vi "itemsLow.vi"(8 "error in (no error)":errorcluster, 11 "reference in":refnum<class "Project Panels.lvclass">=refnum) -> (0 "error out":errorcluster={"status"=TRUE, "code"=1556, "source"="In Place Element Structure in Project Panels.lvclass:items.vi"}, 2 "saved?":bool, 3 "reference out":refnum<class "Project Panels.lvclass">)   [LabVIEW 2015, in "Project Panels.lvclass"]
uses:
  Project Panels.lvclass
  SYS/Items Controller_llb/storageSheets.ctl
  stateItem.ctl
  <vilib>/Utility/miscctls.llb/LVRowAndColumnUnsignedTypeDef.ctl
  <vilib>/Utility/miscctls.llb/LVRowAndColumnTypeDef.ctl
  SYS/Items Controller_llb/Items Controller.lvclass
  SYS/File Controller_llb/File Controller.lvclass
panel:
  out "title":string="Cosmed Asia Pacific - Storage"
  in  "tables":enum32{"Check IN", "Check OUT", "Storage"}(tab)
  in  "checkIN":string[][](table)
  in  "checkOUT":string[][](table)
  in  "Storage":string[][](table)
  in  "uploadFile":bool
  in  "Add Check OUT":bool
  in  "Add Check IN":bool
  out "Number of Items:":i32
  out "index":i32
  in  "back":bool
  in  "next":bool
  out "storageSheets":T1
  in  "Search Item":bool
  in  "Save":bool
  out "Item Selected (S/N or P/N):":string
  out "statuBar":string="Stoped for an Error"
  in  "Stop Button":bool
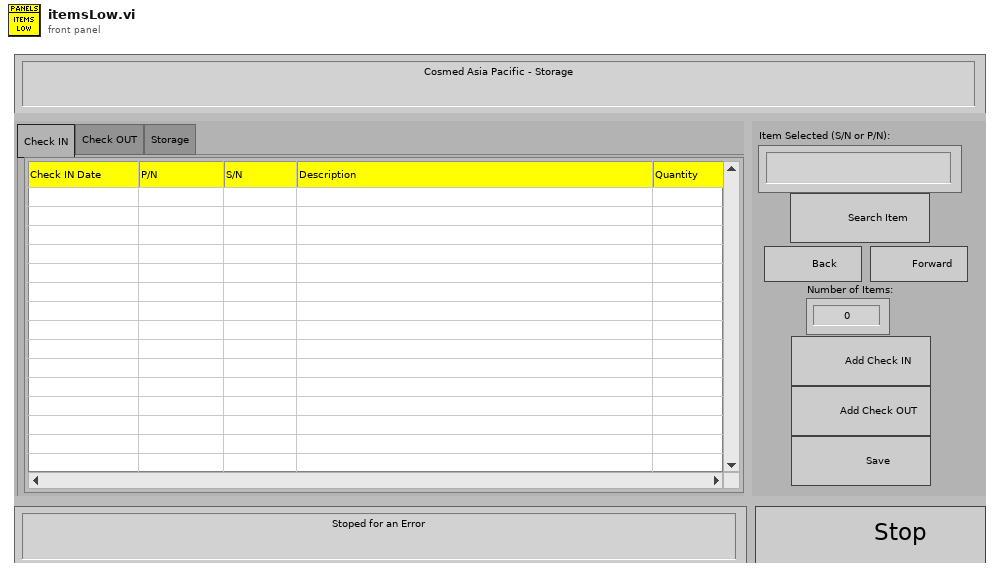
[diagram p1: front panel]
types:
  T1 = typedef "Items Controller.lvclass/storageSheets.ctl" = enum16{"check-in", "check-out", "storage"}
  T2 = typedef "Project Panels.lvclass/stateItem.ctl" = enum16{"initiate", "waitEvent", "save", "search", "UploadFile", "nextItems", "stop"}
  T3 = typedef "LVRowAndColumnUnsignedTypeDef.ctl" = cluster{"Row":u32, "Column":u32}
  T4 = enum8{"Enabled", "Disabled", "Disabled and Grayed Out"}
  T5 = cluster{"checkIN":string[][], "checkOUT":string[][], "storage":string[][]}
  T6 = typedef "LVRowAndColumnTypeDef.ctl" = cluster{"Row":i32, "Column":i32}
  T7 = typedef "Project Panels.lvclass/ObjectAttributesRef.ctl" = refnum<data-value>
  T8 = typedef "Project Panels.lvclass/ObjectAttributes.ctl" = cluster{"MyAttribute":dbl, "device_controller_ref":refnum<class "Devices Controller.lvclass">, "file_controller_ref":refnum<class "File Controller.lvclass">, "item_controller_ref":refnum<class "Items Controller.lvclass">, "item_tables":cluster{"checkIN":string[][], "checkOUT":string[][], "storage":string[][]}, "quickbook_table":cluster{"notes":string[][]}, "notification_controller_ref":refnum<class "Notification Controller.lvclass">, "partstracking_controller_ref":refnum<class "PartsTracking Controller.lvclass">, "product_tables":cluster{"k4b2":string[][], "fitmate":string[][], "RMR":string[][], "CPET":string[][], "BP":string[][], "PP":string[][], "k5":string[][], "bb-pft":string[][]}, "rowsColour":u32[], "low_resolution?":bool, "run_python?":bool}
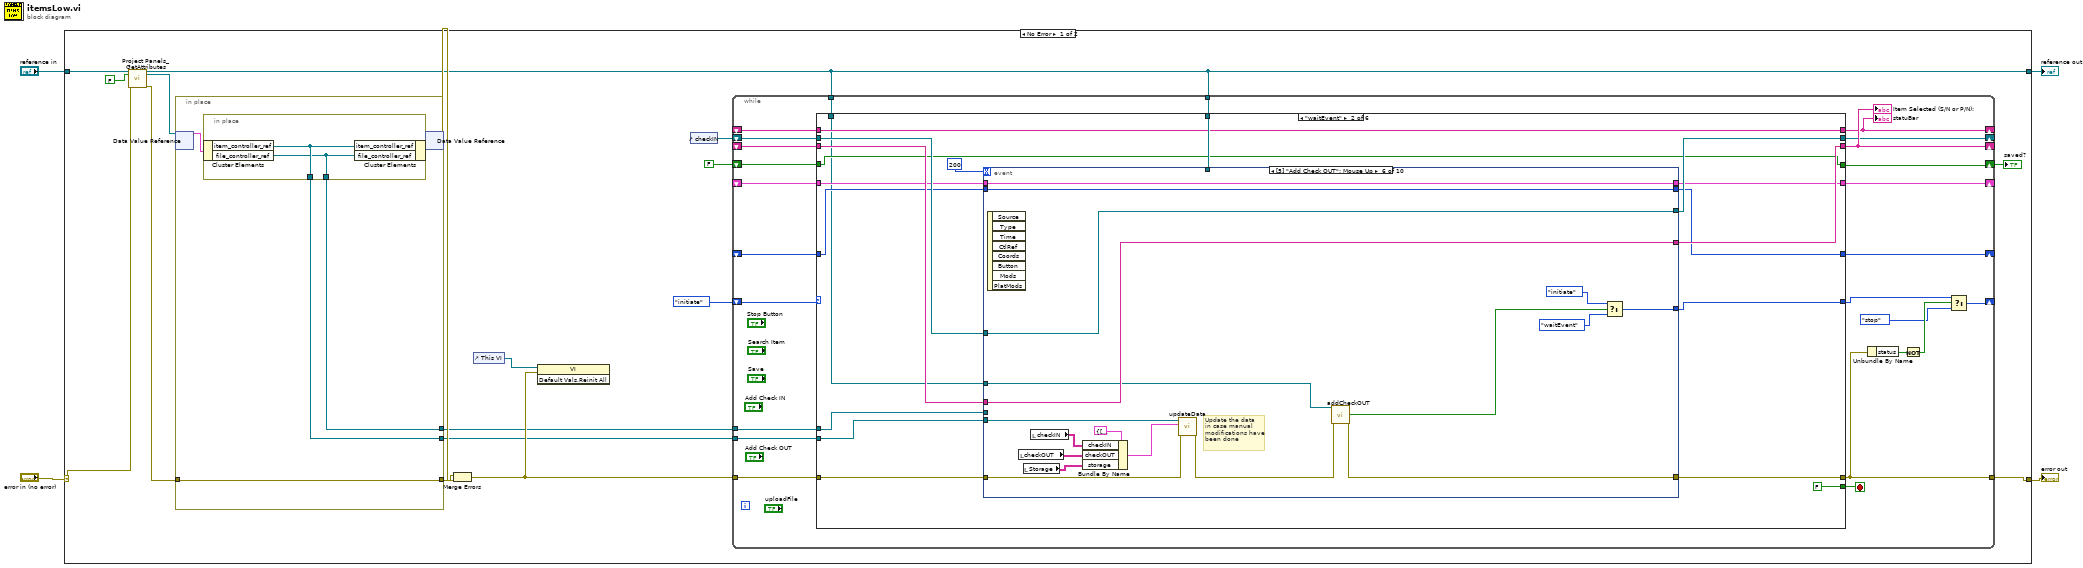
[diagram p0: block diagram]
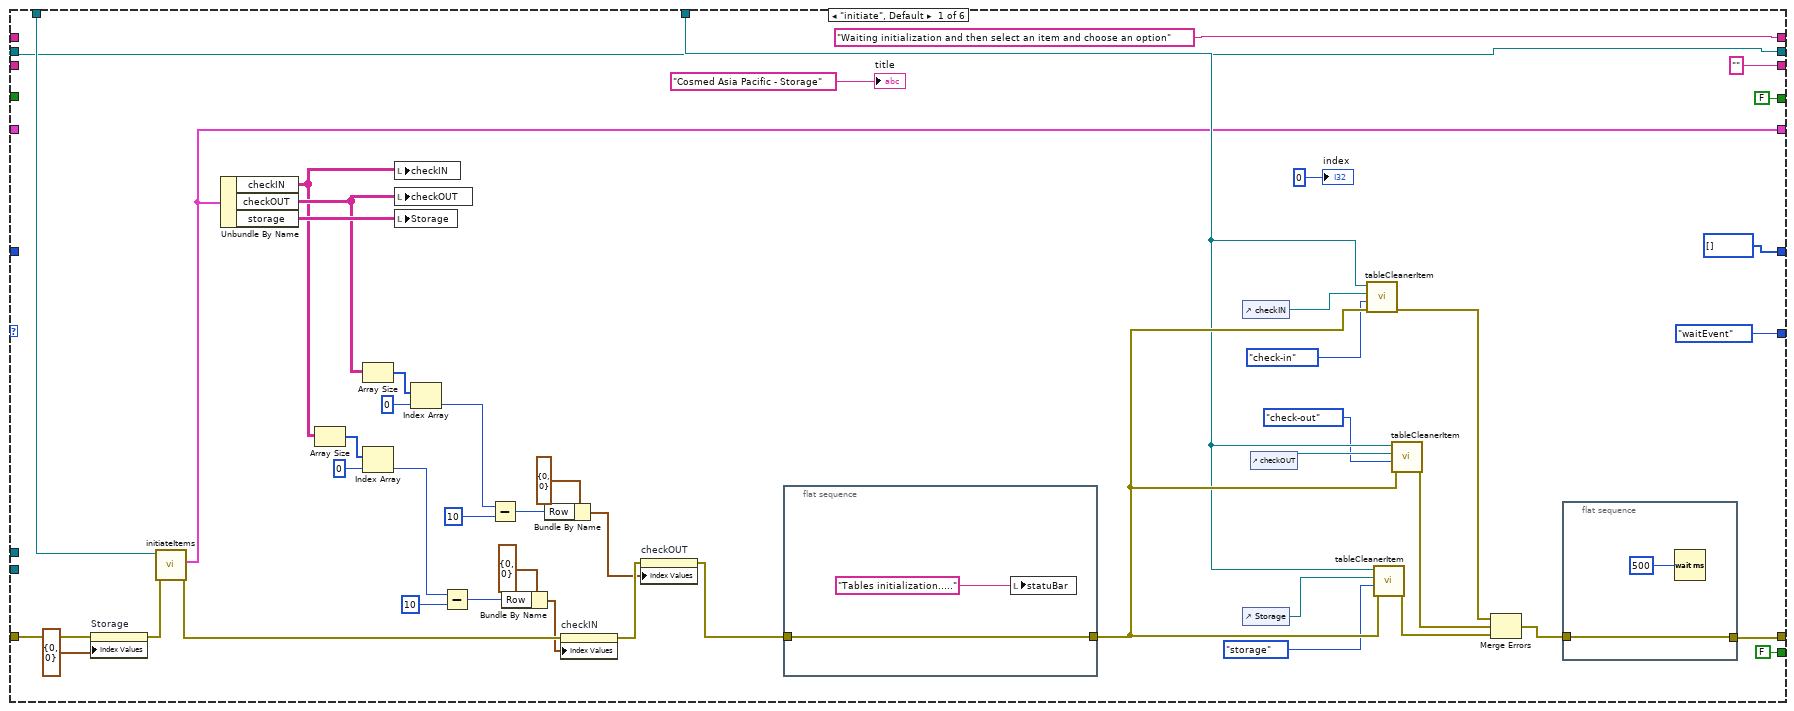
[diagram p2: hidden frame]
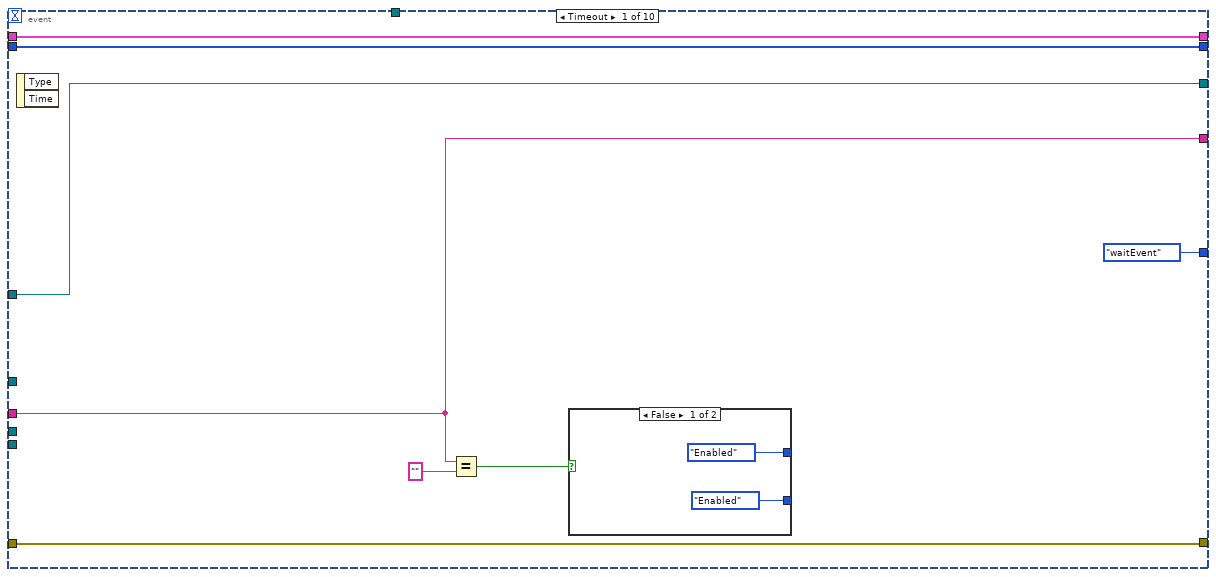
[diagram p3: hidden frame]
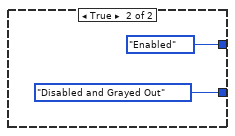
[diagram p4: hidden frame]
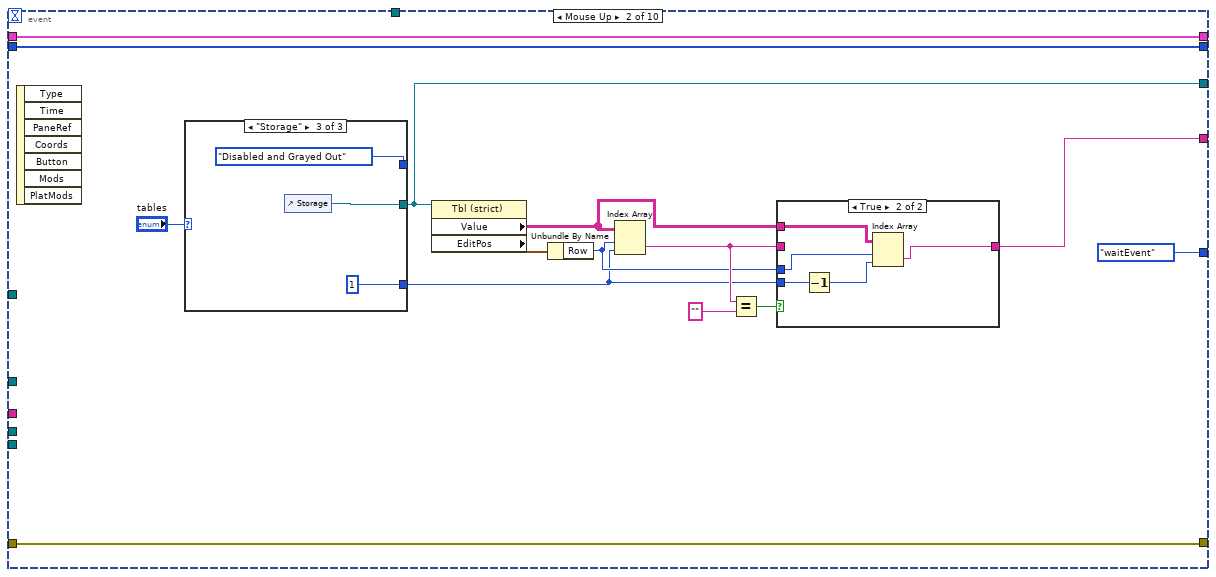
[diagram p5: hidden frame]
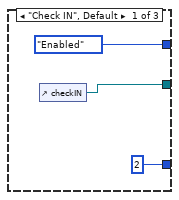
[diagram p7: hidden frame]
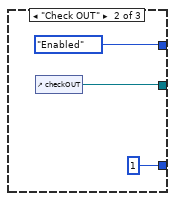
[diagram p8: hidden frame]
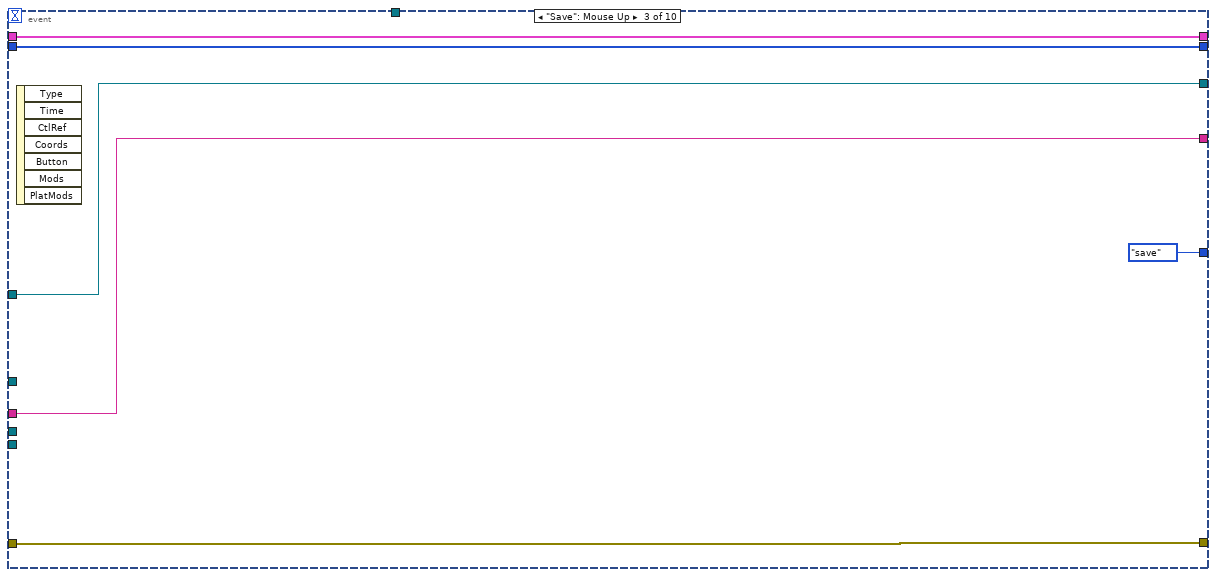
[diagram p9: hidden frame]
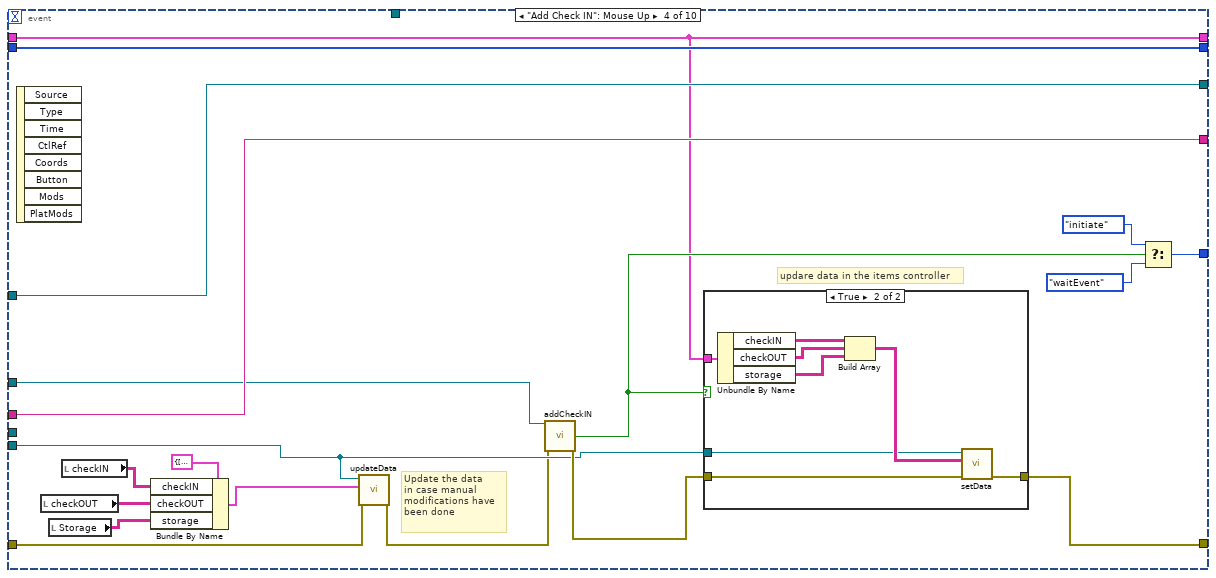
[diagram p10: hidden frame]
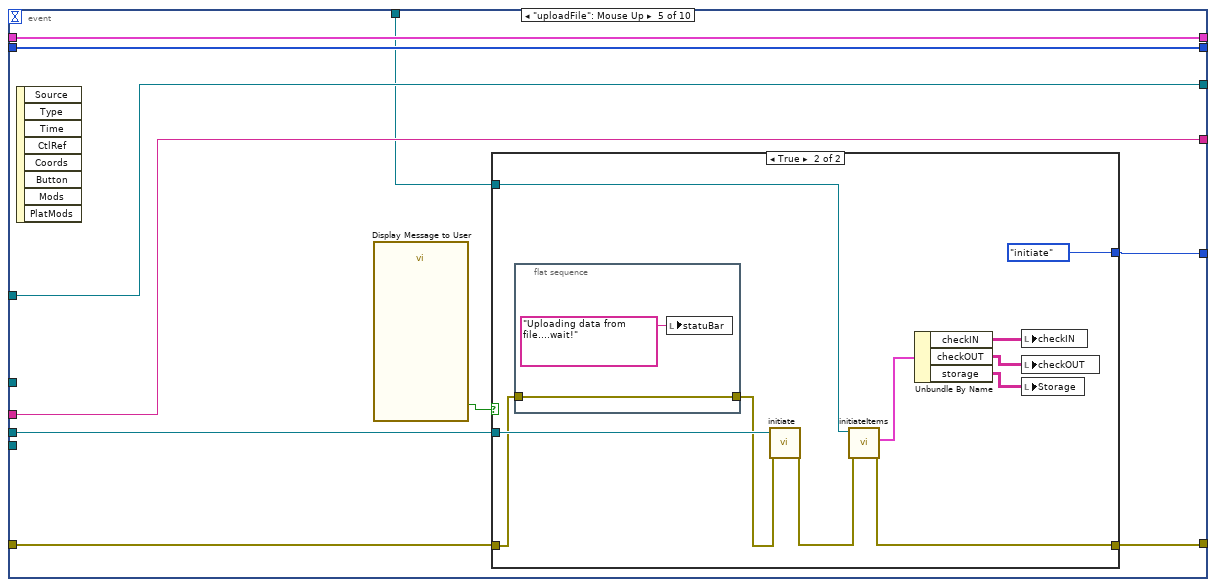
[diagram p12: hidden frame]
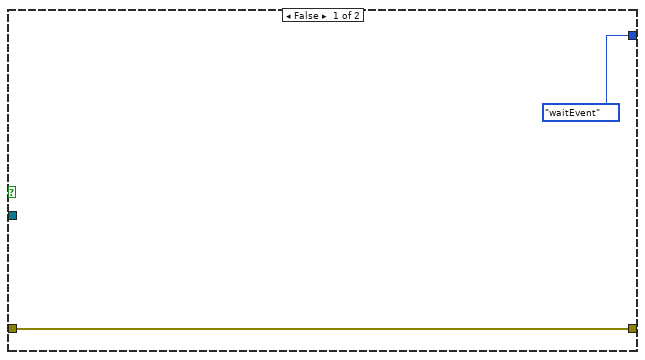
[diagram p13: hidden frame]
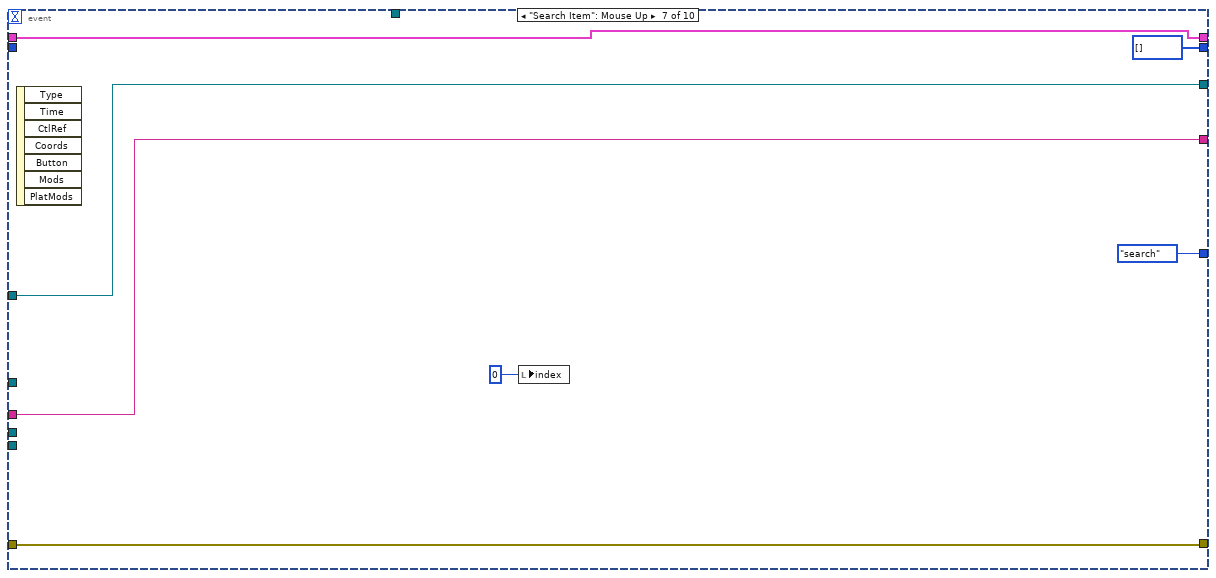
[diagram p14: hidden frame]
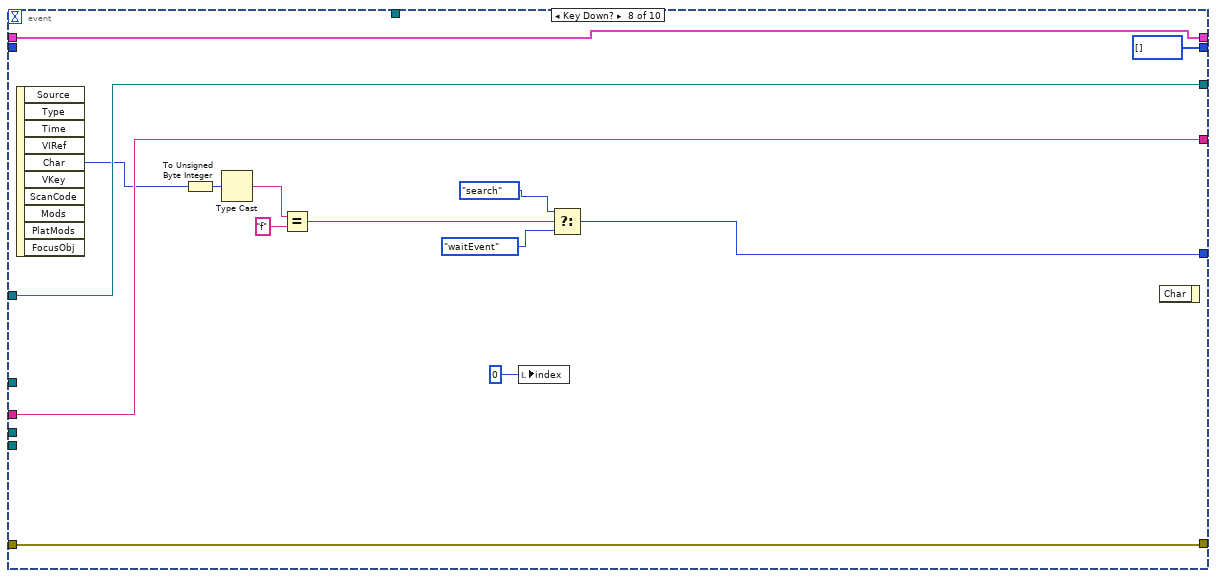
[diagram p15: hidden frame]
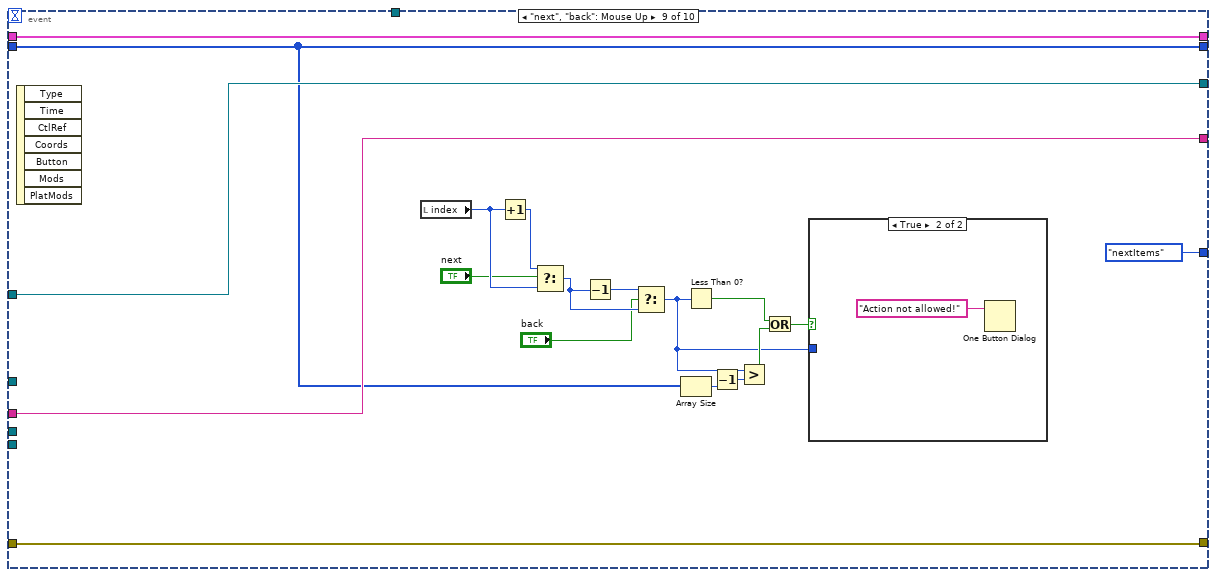
[diagram p16: hidden frame]
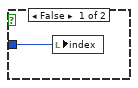
[diagram p17: hidden frame]
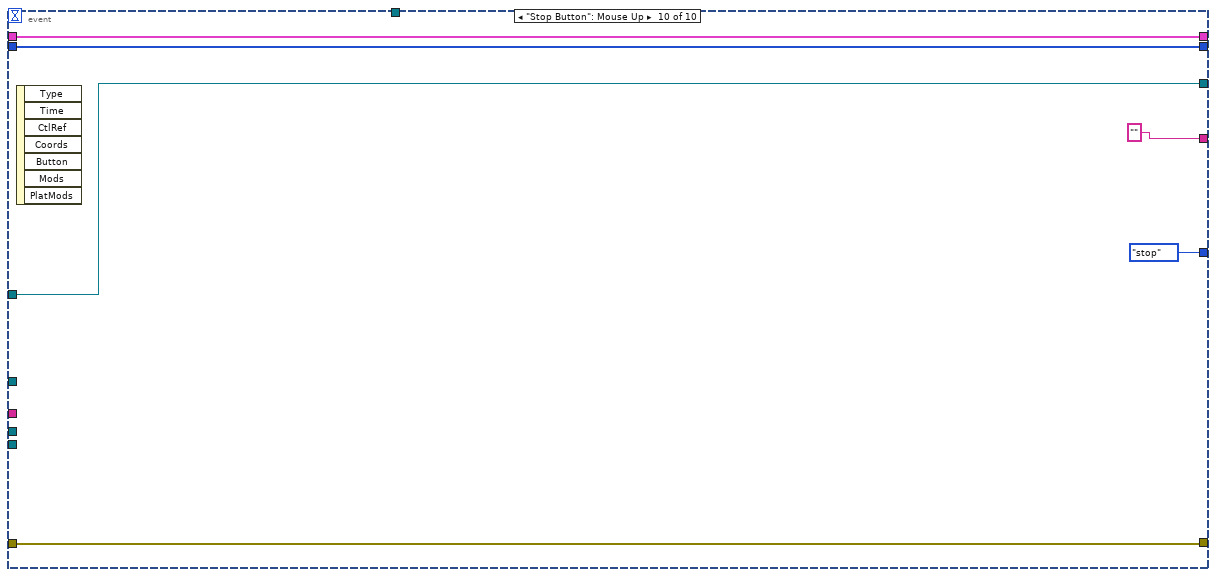
[diagram p18: hidden frame]
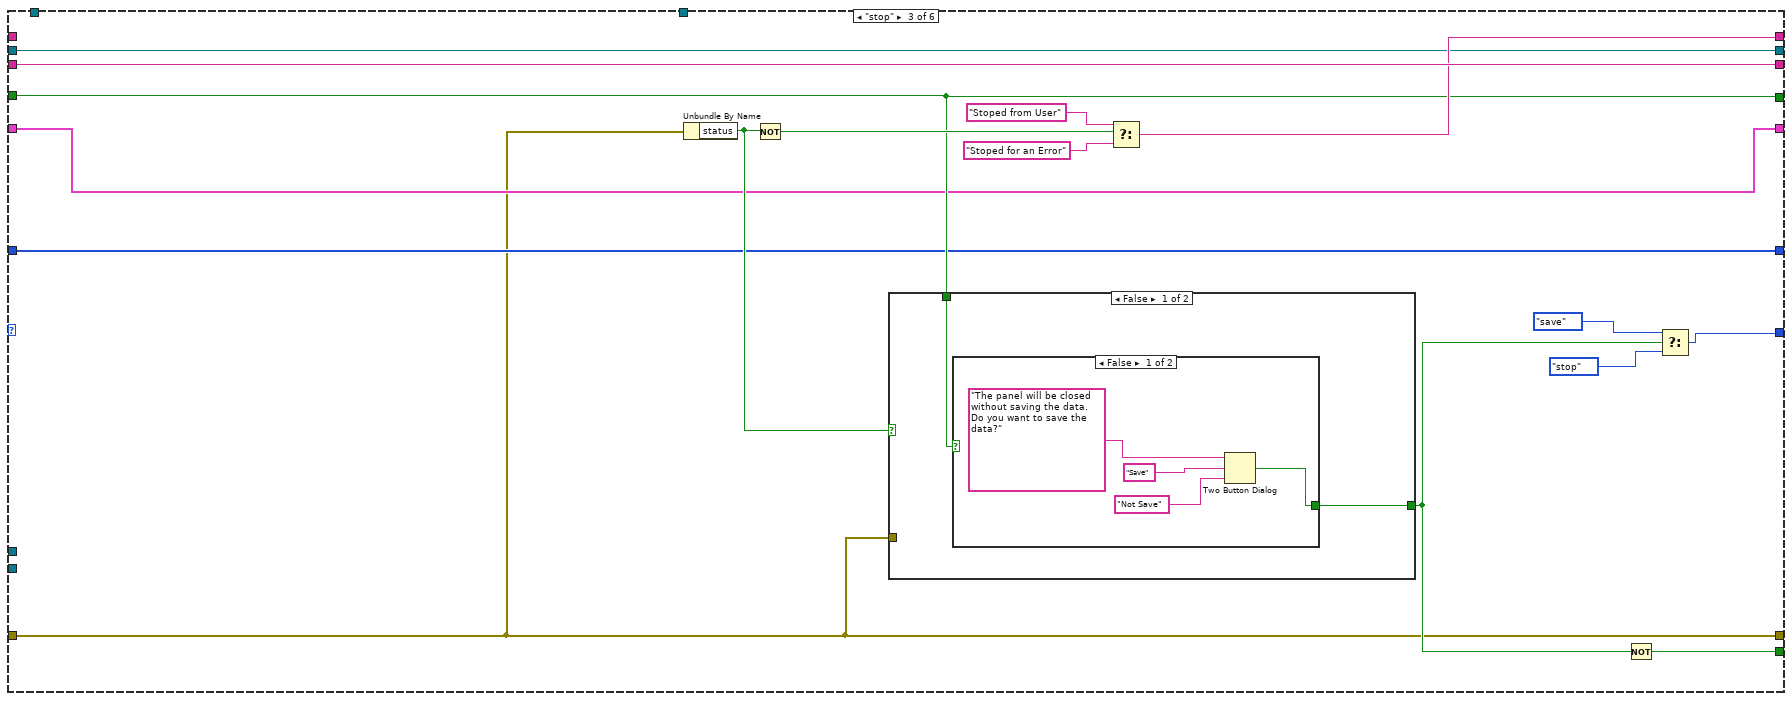
[diagram p19: hidden frame]
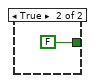
[diagram p20: hidden frame]
diagram:
  n1 = case shown="No Error" "error in (no error)" {
    selector: "error in (no error)" -> [w17 w412]
    tunnel: [w14 w412] -> w3
    tunnel: [w12 w411] -> w1
    tunnel: "reference in" -> [w19 w411]
    frame No Error {
      n2 = call "Project Panels_GetAttributes.vi"("reference in"=w19, "return data? (T)"=FALSE, "error in (no error)"=w17) -> ("reference out"=w12:refnum<class "Project Panels.lvclass">, "attributes ref"=w15:T7, "error out"=w16:errorcluster)  [unwired: 13 in, 1 out]
      n3 = in-place {
        in-place-border: w16 -> [w406]
        in-place-border: [w406] -> w20
        in-place-border: [w405] -> w8
        in-place-border: [w404] -> w5
        n4 = in-place-dvr #1(w15) -> (w407:T8)  [unwired: 1 out]
        n5 = in-place {
          in-place-border: [w410] -> w405
          in-place-border: [w409] -> w404
          n6 = in-place-cluster #2(w407) -> ("item_controller_ref"=w410:refnum<class "Items Controller.lvclass">, "file_controller_ref"=w409:refnum<class "File Controller.lvclass">)
          n7 = in-place-cluster #2("item_controller_ref"=w410, "file_controller_ref"=w409) -> (w408:T8)
        }
        n8 = in-place-dvr #1(w408) -> (w21:errorcluster)  [unwired: 1 out]
      }
      n9 = Merge Errors(w20, w21) -> (w9:errorcluster)
      n10 = control-ref of="This VI"() -> (w10:refnum<vi>)
      n11 = invoke class="VI" method="Default Vals.Reinit All"(reference=w10, error in=w9) -> ()  [unwired: 1 in, 3 out]
      n12 = control-ref of="checkIN"() -> (w11:refnum<vi>)
      n13 = while {
        tunnel: w12 -> [w46]
        tunnel: w9 -> [w45]
        tunnel: [w43] -> w14
        shift-right: [w40] -> _
        shift-left: stateItem."initiate" ("state") -> [w44]
        shift-right: [w37] -> _
        shift-left: _ -> [w36]
        shift-right: [w35] -> _
        shift-left: w11 -> [w34]
        tunnel: w12 -> [w33]
        tunnel: w8 -> [w31]
        shift-right: [w29] -> w6
        shift-left: FALSE -> [w30]
        shift-right: [w28] -> _
        shift-left: _ -> [w27]
        shift-right: [w26] -> _
        shift-left: _ -> [w25]
        shift-right: [w24] -> _
        shift-left: _ -> [w23]
        tunnel: w5 -> [w22]
        stop <- w38 stop-if-true
        n14 = case shown="\"waitEvent\"" w44 {
          tunnel: w46 -> [w81 w106 _ _ _ _]
          tunnel: w45 -> [w74 w115 w282 w310 w342 w377]
          tunnel: [w84 w109 w282 w321 w342 w373] -> w43
          tunnel: [stateItem."waitEvent" ("state") w108 w288 w316 stateItem."waitEvent" ("state") stateItem."waitEvent" ("state")] -> w41
          tunnel: [FALSE FALSE w287 FALSE FALSE FALSE] -> w38
          tunnel: ["Waiting initialization and then select an item and choose an option" ("title") w104 w294 "Search Item option selected..." ("title") "Click on the arrows to select other items" ("title") w372] -> w28
          tunnel: ["" w111 w297 w322 w339 w378] -> w37
          tunnel: w36 -> [_ w113 w297 w322 w339 w378]
          tunnel: [w78 w110 w293 w323 w333 w379] -> w35
          tunnel: w34 -> [w78 w112 w293 w323 w333 w379]
          tunnel: w33 -> [w80 w99 _ w312 _ _]
          tunnel: w31 -> [_ w107 _ _ _ w350]
          tunnel: w30 -> [_ w105 w286 w320 w340 _]
          tunnel: [FALSE w105 w286 w320 w340 TRUE] -> w29
          tunnel: w27 -> [_ w104 _ _ _ _]
          tunnel: [i32[] [] ("indexElements") w102 w285 w314 w334 w375] -> w26
          tunnel: w25 -> [_ w103 w285 _ w334 w375]
          tunnel: [w47 w100 w284 w311 w326 w371] -> w24
          tunnel: w23 -> [_ w101 w284 w311 w326 w371]
          tunnel: w22 -> [_ w98 _ _ _ _]
          frame "initiate", Default {
            n15 = property on="Storage" class="Tbl (strict)"(error in=w74, "Index Values"=T3 {"Row"=0, "Column"=0}) -> (error out=w73:errorcluster)  [unwired: 1 in, 1 out]
            n16 = call "initiateItems.vi"("error in (no error)"=w73, "reference in"=w80) -> ("error out"=w65:errorcluster, "table"=w47:T5)  [unwired: 7 in, 1 out]
            n17 = Unbundle By Name(w47) -> ("checkIN"=w48:string[][], "checkOUT"=w67:string[][], "storage"=w72:string[][])
            n18 = Array Size(array=w48) -> (size(s)=w54:i32[])
            n19 = Array Size(array=w67) -> (size(s)=w61:i32[])
            n20 = Index Array(array=w54, index=0) -> (element=w51:i32)
            n21 = local write "checkIN"(w48) -> ()
            n22 = local write "checkOUT"(w67) -> ()
            n23 = local write "Storage"(w72) -> ()
            n24 = Index Array(array=w61, index=0) -> (element=w58:i32)
            n25 = Subtract(x=w51, y=10) -> (x-y=w52:i32)
            n26 = Subtract(x=w58, y=10) -> (x-y=w59:i32)
            n27 = Bundle By Name(cluster=T3 {"Row"=0, "Column"=0} ("Index Values"), "Row"=w52) -> (w49:T3)
            n28 = Bundle By Name(cluster=T3 {"Row"=0, "Column"=0} ("Index Values"), "Row"=w59) -> (w56:T3)
            n29 = property on="checkIN" class="Tbl (strict)"(error in=w65, "Index Values"=w49) -> (error out=w64:errorcluster)  [unwired: 1 in, 1 out]
            n30 = property on="checkOUT" class="Tbl (strict)"(error in=w64, "Index Values"=w56) -> (error out=w66:errorcluster)  [unwired: 1 in, 1 out]
            n31 = flat-sequence {
              tunnel: w66 -> [w95]
              tunnel: [w95] -> w83
              frame #0 {
                n32 = local write "statuBar"("Tables initialization....." ("title")) -> ()
              }
            }
            n33 = control-ref of="checkIN"() -> (w91:refnum<vi>)
            n34 = control-ref of="Storage"() -> (w93:refnum<vi>)
            n35 = control-ref of="checkOUT"() -> (w92:refnum<vi>)
            n36 = call "tableCleanerItem.vi"("error in (no error)"=w83, "storageSheets"=storageSheets."check-in", "Table in"=w91, "reference in"=w81) -> ("error out"=w90:errorcluster)  [unwired: 6 in, 1 out]
            n37 = call "tableCleanerItem.vi"("error in (no error)"=w83, "storageSheets"=storageSheets."storage", "Table in"=w93, "reference in"=w81) -> ("error out"=w88:errorcluster)  [unwired: 6 in, 1 out]
            n38 = call "tableCleanerItem.vi"("error in (no error)"=w83, "storageSheets"=storageSheets."check-out", "Table in"=w92, "reference in"=w81) -> ("error out"=w89:errorcluster)  [unwired: 6 in, 1 out]
            n39 = Merge Errors(w90, w89, w88) -> (w79:errorcluster)
            n40 = flat-sequence {
              tunnel: w79 -> [w97]
              tunnel: [w97] -> w84
              frame #0 {
                n41 = Wait (ms)(milliseconds to wait=u32 500) -> ()  [unwired: 1 out]
              }
            }
            "title" <- "Cosmed Asia Pacific - Storage" ("title")
            "index" <- 0 ("index")
          }
          frame "waitEvent" {
            n42 = event shown="[5] \"Add Check OUT\": Mouse Up" {
              selector: _ -> [_ _ _ _ _ _ _ _ _ _]
              dyn-events: _ -> [_ _ _ _ _ _ _ _ _ _]
              timeout: 200 -> [_ _ _ _ _ _ _ _ _ _]
              tunnel: w115 -> [w124 w142 w158 w170 w197 w225 w238 w253 w273 w281]
              tunnel: [w124 w142 w158 w173 w196 w230 w238 w253 w273 w281] -> w109
              tunnel: w113 -> [w120 _ w162 w182 w198 w234 w240 w254 w266 _]
              tunnel: w112 -> [w121 _ w163 w181 w199 w233 w241 w255 w267 w279]
              tunnel: [w120 w135 w162 w182 w198 w234 w240 w254 w266 ""] -> w111
              tunnel: [w121 w139 w163 w181 w199 w233 w241 w255 w267 w279] -> w110
              tunnel: [stateItem."waitEvent" ("state") stateItem."waitEvent" ("state") stateItem."save" ("state") w177 w194 w228 stateItem."search" ("state") w243 stateItem."nextItems" ("state") stateItem."stop" ("state")] -> w108
              tunnel: w107 -> [_ _ _ w172 _ w223 _ _ _ _]
              tunnel: w106 -> [_ _ _ _ w192 _ _ _ _ _]
              tunnel: w103 -> [w118 w130 w160 w180 w200 w232 _ _ w265 w277]
              tunnel: [w118 w130 w160 w180 w200 w232 i32[] [] ("indexElements") i32[] [] ("indexElements") w265 w277] -> w102
              tunnel: w101 -> [w117 w129 w159 w171 w201 w222 w235 w250 w256 w276]
              tunnel: [w117 w129 w159 w171 w201 w222 w235 w250 w256 w276] -> w100
              tunnel: w99 -> [_ _ _ w179 _ w231 _ _ _ _]
              tunnel: w98 -> [_ _ _ _ w193 _ _ _ _ _]
              event Timeout {
                n43 = event-data() -> ()  [unwired: 1 in, 2 out]
                n44 = Equal?(x=w120, y="") -> (x = y?=w123:bool)
                n45 = case shown="False" w123 {
                  tunnel: [T4."Enabled" ("Disabled") T4."Disabled and Grayed Out" ("Disabled")] -> _
                  tunnel: [T4."Enabled" ("Disabled") T4."Enabled" ("Disabled")] -> _
                  frame False {
                  }
                  frame True {
                  }
                }
              }
              event Mouse Up {
                n46 = event-data() -> ()  [unwired: 1 in, 7 out]
                n47 = case shown="\"Storage\"" "tables" {
                  tunnel: [w151 w154 w157] -> w139
                  tunnel: [T4."Enabled" ("Disabled") T4."Enabled" ("Disabled") T4."Disabled and Grayed Out" ("Disabled")] -> _
                  tunnel: [2 ("disabled index (col)") 1 ("disabled index (col)") 1 ("disabled index (col)")] -> w132
                  frame "Check IN", Default {
                    n48 = control-ref of="checkIN"() -> (w151:refnum<vi>)
                  }
                  frame "Check OUT" {
                    n49 = control-ref of="checkOUT"() -> (w154:refnum<vi>)
                  }
                  frame "Storage" {
                    n50 = control-ref of="Storage"() -> (w157:refnum<vi>)
                  }
                }
                n51 = property on="Property Node" class="Tbl (strict)"(reference=w139) -> ("Value"=w134:string[][], "EditPos"=w141:T6)  [unwired: 1 in, 2 out]
                n52 = Unbundle By Name(w141) -> ("Row"=w133:i32)
                n53 = Index Array(array=w134, index (row)=w133, index (col)=w132) -> (element=w136:string)
                n54 = Equal?(x=w136, y="") -> (x = y?=w137:bool)
                n55 = case shown="True" w137 {
                  tunnel: w136 -> [w143 _]
                  tunnel: [w143 w144] -> w135
                  tunnel: w134 -> [_ w148]
                  tunnel: w133 -> [_ w147]
                  tunnel: w132 -> [_ w146]
                  frame False {
                  }
                  frame True {
                    n56 = Decrement(x=w146) -> (x-1=w145:i32)
                    n57 = Index Array(array=w148, index (row)=w147, index (col)=w145) -> (element=w144:string)
                  }
                }
              }
              event "Save": Mouse Up {
                n58 = event-data() -> ()  [unwired: 1 in, 7 out]
              }
              event "Add Check IN": Mouse Up {
                # "Update the data\nin case manual\nmodifications have\nbeen done"
                # "updare data in the items controller"
                n59 = event-data() -> ()  [unwired: 1 in, 8 out]
                n60 = local read "checkOUT"() -> (w166:string[][])
                n61 = local read "Storage"() -> (w165:string[][])
                n62 = local read "checkIN"() -> (w167:string[][])
                n63 = Bundle By Name(cluster=T5 {"checkIN"=[], "checkOUT"=[], "storage"=[]} ("table"), "checkIN"=w167, "checkOUT"=w166, "storage"=w165) -> (w164:T5)
                n64 = call "updateData.vi"("error in (no error)"=w170, "table"=w164, "reference in"=w172) -> ("error out"=w169:errorcluster)  [unwired: 7 in, 1 out]
                n65 = call "addCheckIN.vi"("reference in"=w179, "error in (no error)"=w169) -> ("saved?"=w175:bool, "error out"=w174:errorcluster)  [unwired: 11 in, 1 out]
                n66 = case shown="True" w175 {
                  tunnel: w171 -> [_ w187]
                  tunnel: w174 -> [w183 w186]
                  tunnel: [w183 w185] -> w173
                  tunnel: w172 -> [_ w184]
                  frame False {
                  }
                  frame True {
                    n67 = Unbundle By Name(w187) -> ("checkIN"=w191:string[][], "checkOUT"=w190:string[][], "storage"=w189:string[][])
                    n68 = Build Array(w191, w190, w189) -> (w188:string[][][])
                    n69 = call "setData.vi"("error in (no error)"=w186, "data"=w188, "reference in"=w184) -> ("error out"=w185:errorcluster)  [unwired: 7 in, 1 out]
                  }
                }
                n70 = Select(t=stateItem."initiate" ("state"), s=w175, f=stateItem."waitEvent") -> (s? t:f=w177:T2)
              }
              event "uploadFile": Mouse Up {
                n71 = event-data() -> ()  [unwired: 1 in, 8 out]
                n72 = call "Display Message to User"() -> ("Yes"=w195:bool)  [unwired: 10 in, 1 out]
                n73 = case shown="True" w195 {
                  tunnel: w197 -> [w203 w205]
                  tunnel: [w203 w209] -> w196
                  tunnel: [stateItem."waitEvent" ("state") stateItem."initiate" ("state")] -> w194
                  tunnel: w193 -> [_ w213]
                  tunnel: w192 -> [_ w211]
                  frame False {
                  }
                  frame True {
                    n74 = flat-sequence {
                      tunnel: w205 -> [w216]
                      tunnel: [w216] -> w204
                      frame #0 {
                        n75 = local write "statuBar"("Uploading data from file....wait!" ("statuBar")) -> ()
                      }
                    }
                    n76 = call "initiate.vi"("reference in"=w213, "error in (no error)"=w204) -> ("error out"=w210:errorcluster)  [unwired: 16 in, 1 out]
                    n77 = call "initiateItems.vi"("error in (no error)"=w210, "reference in"=w211) -> ("error out"=w209:errorcluster, "table"=w212:T5)  [unwired: 7 in, 1 out]
                    n78 = Unbundle By Name(w212) -> ("checkIN"=w208:string[][], "checkOUT"=w207:string[][], "storage"=w206:string[][])
                    n79 = local write "checkIN"(w208) -> ()
                    n80 = local write "checkOUT"(w207) -> ()
                    n81 = local write "Storage"(w206) -> ()
                  }
                }
              }
              event "Add Check OUT": Mouse Up {
                # "Update the data\nin case manual\nmodifications have\nbeen done"
                n82 = event-data() -> ()  [unwired: 1 in, 8 out]
                n83 = local read "checkOUT"() -> (w219:string[][])
                n84 = local read "Storage"() -> (w218:string[][])
                n85 = local read "checkIN"() -> (w220:string[][])
                n86 = Bundle By Name(cluster=T5 {"checkIN"=[], "checkOUT"=[], "storage"=[]} ("table"), "checkIN"=w220, "checkOUT"=w219, "storage"=w218) -> (w217:T5)
                n87 = call "updateData.vi"("error in (no error)"=w225, "table"=w217, "reference in"=w223) -> ("error out"=w224:errorcluster)  [unwired: 7 in, 1 out]
                n88 = call "addCheckOUT.vi"("reference in"=w231, "error in (no error)"=w224) -> ("saved?"=w227:bool, "error out"=w230:errorcluster)  [unwired: 11 in, 1 out]
                n89 = Select(t=stateItem."initiate" ("state"), s=w227, f=stateItem."waitEvent") -> (s? t:f=w228:T2)
              }
              event "Search Item": Mouse Up {
                n90 = event-data() -> ()  [unwired: 1 in, 7 out]
                n91 = local write "index"(0 ("index")) -> ()
              }
              event Key Down? {
                n92 = event-data() -> ("Char"=w248:i16)  [unwired: 1 in, 9 out]
                n93 = To Unsigned Byte Integer(number=w248) -> (unsigned 8bit integer=w249:u8)
                n94 = Type Cast(x=w249) -> (*(type *) &x=w247:string)  [unwired: 1 in]
                n95 = Equal?(x=w247, y="f") -> (x = y?=w242:bool)
                n96 = local write "index"(0 ("index")) -> ()
                n97 = Select(t=stateItem."search" ("state"), s=w242, f=stateItem."waitEvent" ("state")) -> (s? t:f=w243:T2)
                n98 = event-data() -> ()  [unwired: 2 in, 1 out]
              }
              event "next", "back": Mouse Up {
                n99 = event-data() -> ()  [unwired: 1 in, 7 out]
                n100 = local read "index"() -> (w271:i32)
                n101 = Increment(x=w271) -> (x+1=w272:i32)
                n102 = Select(t=w272, s="next", f=w271) -> (s? t:f=w269:i32)
                n103 = Decrement(x=w269) -> (x-1=w270:i32)
                n104 = Select(t=w270, s="back", f=w269) -> (s? t:f=w260:i32)
                n105 = Array Size(array=w265) -> (size(s)=w264:i32)
                n106 = Less Than 0?(x=w260) -> (x < 0?=w262:bool)
                n107 = Decrement(x=w264) -> (x-1=w257:i32)
                n108 = Greater?(x=w260, y=w257) -> (0:w263:bool)
                n109 = Or(x=w262, y=w263) -> (x .or. y?=w261:bool)
                n110 = case shown="True" w261 {
                  tunnel: w260 -> [w274 _]
                  frame False {
                    n111 = local write "index"(w274) -> ()
                  }
                  frame True {
                    n112 = One Button Dialog(message="Action not allowed!") -> ()  [unwired: 1 in, 1 out]
                  }
                }
              }
              event "Stop Button": Mouse Up {
                n113 = event-data() -> ()  [unwired: 1 in, 7 out]
              }
            }
          }
          frame "stop" {
            n114 = Unbundle By Name(w282) -> ("status"=w292:bool)
            n115 = Not(x=w292) -> (.not. x?=w291:bool)
            n116 = case shown="False" w292 {
              tunnel: w282 -> [_ w307]
              tunnel: [w299 FALSE ("Save")] -> w283
              tunnel: w286 -> [w298 _]
              frame False {
                n117 = case shown="False" w298 {
                  tunnel: [w302 FALSE ("Save")] -> w299
                  frame False {
                    n118 = Two Button Dialog(message="The panel will be closed without saving the data. Do you want to save the data?", 1:"Not Save" ("F button name (\"Cancel\")"), 2:"Save" ("T button name (\"OK\")")) -> (T button?=w302:bool)
                  }
                  frame True {
                  }
                }
              }
              frame True {
                n119 = Unbundle By Name(w307) -> ("source"=w306:string)
                n120 = Concatenate Strings("An Error occur: " ("message"), w306) -> (w309:string)
                n121 = One Button Dialog(message=w309) -> ()  [unwired: 1 in, 1 out]
              }
            }
            n122 = Select(t="Stoped from User" ("title"), s=w291, f="Stoped for an Error" ("title")) -> (s? t:f=w294:string)
            n123 = Not(x=w283) -> (.not. x?=w287:bool)
            n124 = Select(t=stateItem."save", s=w283, f=stateItem."stop" ("state")) -> (s? t:f=w288:T2)
          }
          frame "search" {
            n125 = call "searchItem.vi"("reference in"=w312, "error in (no error)"=w310) -> ("Sheet out"=→"storageSheets":T1, "indexElements"=w314:i32[], "error out"=w321:errorcluster)  [unwired: 10 in, 1 out]
            n126 = Array Size(array=w314) -> (size(s)=w313:i32)
            "Number of Items:" <- w313
            n127 = Greater Than 0?(x=w313) -> (x > 0?=w315:bool)
            n128 = Select(t=stateItem."nextItems" ("state"), s=w315, f=stateItem."waitEvent" ("state")) -> (s? t:f=w316:T2)
          }
          frame "nextItems" {
            n129 = local read "storageSheets"() -> (w329:T1)
            n130 = local read "index"() -> (w336:i32)
            n131 = case shown="\"storage\"" w329 {
              tunnel: [w344 w346 w348] -> w328
              tunnel: [enum32{"Check IN", "Check OUT", "Storage"}."Check IN" ("tables") enum32{"Check IN", "Check OUT", "Storage"}."Check OUT" ("tables") enum32{"Check IN", "Check OUT", "Storage"}."Storage" ("tables")] -> w327
              frame "check-in", Default {
                n132 = control-ref of="checkIN"() -> (w344:refnum<vi>)
              }
              frame "check-out" {
                n133 = control-ref of="checkOUT"() -> (w346:refnum<vi>)
              }
              frame "storage" {
                n134 = control-ref of="Storage"() -> (w348:refnum<vi>)
              }
            }
            n135 = Index Array(array=w334, index=w336) -> (element=w335:i32)
            n136 = Bundle By Name(cluster=T6 {"Row"=0, "Column"=0} ("Active Cell:Active Cell"), "Row"=w335, "Column"=0) -> (w330:T6)
            n137 = local write "tables"(w327) -> ()
            n138 = property on="Property Node" class="Tbl (strict)"(reference=w328, "Index Values"=w330) -> ()  [unwired: 1 in, 2 out]
          }
          frame "save" {
            w362 = 0 ("index")
            n139 = flat-sequence {
              tunnel: w377 -> [w403]
              tunnel: [w403] -> w352
              frame #0 {
                n140 = local write "statuBar"("Saving...wait" ("title")) -> ()
              }
            }
            n141 = Array Size(array="checkIN") -> (size(s)=w365:i32[])
            n142 = Array Size(array="checkOUT") -> (size(s)=w364:i32[])
            n143 = Array Size(array="Storage") -> (size(s)=w363:i32[])
            n144 = Index Array(array=w363, index=w362) -> (element=w359:i32)
            n145 = Index Array(array=w364, index=w362) -> (element=w360:i32)
            n146 = Index Array(array=w365, index=w362) -> (element=w361:i32)
            n147 = Build Array(w361, w360, w359) -> (w358:i32[])
            n148 = Array Max & Min(array=w358) -> (max value=w355:i32)  [unwired: 3 out]
            n149 = Initialize Array("", 3 ("dimension size"), w355, 10 ("dimension size")) -> (w353:string[][][])
            n150 = for {
              N: 3 -> [_]
              shift-right: [w384] -> w369
              shift-left: w353 -> [w386]
              tunnel: "checkIN" -> [w385]
              tunnel: "checkOUT" -> [w383]
              tunnel: "Storage" -> [w382]
              i -> [w387]
              n151 = case shown="2" w387 {
                tunnel: w386 -> [w391 w395 w399]
                tunnel: w385 -> [w388 _ _]
                tunnel: [w390 w394 w398] -> w384
                tunnel: w383 -> [_ w392 _]
                tunnel: w382 -> [_ _ w396]
                frame 0, Default {
                  n152 = Insert Into Array(array=w391, index (dim 0)=0 ("index (page)"), new element=w388) -> (w390:string[][][])  [unwired: 2 in]
                }
                frame 1 {
                  n153 = Insert Into Array(array=w395, index (dim 0)=1 ("disabled index (page)"), new element=w392) -> (w394:string[][][])  [unwired: 2 in]
                }
                frame 2 {
                  n154 = Insert Into Array(array=w399, index (dim 0)=2 ("disabled index (page)"), new element=w396) -> (w398:string[][][])  [unwired: 2 in]
                }
              }
            }
            n155 = call "setData.vi"("error in (no error)"=w352, "data"=w369, "reference in"=w350) -> ("error out"=w351:errorcluster, "reference out"=w349:refnum<class "Items Controller.lvclass">)  [unwired: 7 in]
            n156 = call "saveData.vi"("error in (no error)"=w351, "reference in"=w349) -> ("error out"=w374:errorcluster)  [unwired: 8 in, 1 out]
            n157 = flat-sequence {
              tunnel: w374 -> [w401]
              tunnel: [w401] -> w373
              tunnel: ["select an item and choose an option" ("title")] -> w372
              frame #0 {
              }
            }
          }
        }
        "statuBar" <- w28
        "Item Selected (S/N or P/N):" <- w37
        n158 = Unbundle By Name(w43) -> ("status"=w42:bool)
        n159 = Not(x=w42) -> (.not. x?=w39:bool)
        n160 = Select(t=w41, s=w39, f=stateItem."stop" ("state")) -> (s? t:f=w40:T2)
      }
      "saved?" <- w6
    }
    frame Error {
    }
  }
  "error out" <- w3
  "reference out" <- w1
